vi "Retrieve CD dependencies from properties.vi"(11 "main page properties in":T5) -> (2 "custom device dependencies":T1[](array[typedef]), 3 "main page properties out":T5)   [LabVIEW 2019, in "HLA Custom Device System Explorer.lvlib"]
uses:
  HLA Custom Device System Explorer.lvlib
  Shared/main_page_config.ctl
  <vilib>/NI VeriStand/Custom Device API/Custom Device File Dependency.ctl
  <vilib>/NI VeriStand/Custom Device API/Path Specification.ctl
  <vilib>/NI VeriStand/Custom Device API/Path Type.ctl
  <vilib>/NI VeriStand/Custom Device API/Custom Device Supported Target.ctl
  Shared/HLA Custom Device Shared.lvlib
  <vilib>/NI VeriStand/Custom Device API/Custom Device API.lvlib
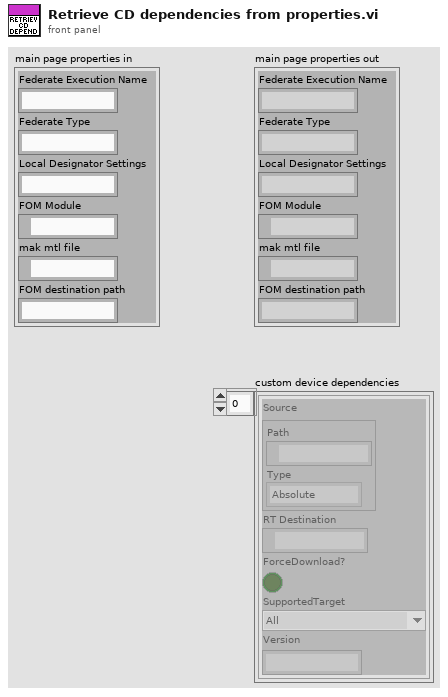
[diagram p1: front panel]
types:
  T1 = typedef "Custom Device API.lvlib/Custom Device File Dependency.ctl" = cluster{"Source":T2, "RT Destination":path, "ForceDownload?":bool, "SupportedTarget":T4, "Version":string}
  T2 = typedef "Custom Device API.lvlib/Path Specification.ctl" = cluster{"Path":path, "Type":T3}
  T3 = typedef "Custom Device API.lvlib/Path Type.ctl" = enum16{"Absolute", "To Base", "To Common Data Dir", "To Application Data Dir"}
  T4 = typedef "Custom Device API.lvlib/Custom Device Supported Target.ctl" = enum16{"All", "PharLap", "VxWorks", "Windows", "Linux_32_ARM", "Linux_x64", "PharLap & Windows", "PharLap & VxWorks", "VxWorks & Windows"}
  T5 = typedef "HLA Custom Device Shared.lvlib/main_page_config.ctl" = cluster{"Federate Execution Name":string, "Federate Type":string, "Local Designator Settings":string, "FOM Module":path, "mak mtl file":path, "FOM destination path":string}
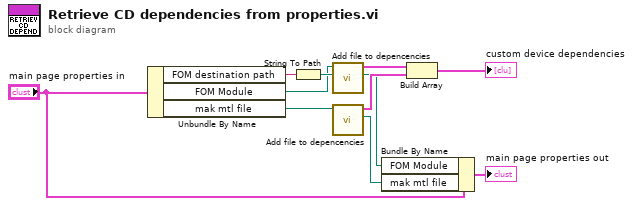
[diagram p0: block diagram]
diagram:
  n1 = Unbundle By Name("main page properties in") -> ("FOM destination path"=w11:string, "FOM Module"=w1:path, "mak mtl file"=w9:path)
  n2 = String To Path(string=w11) -> (path=w10:path)
  n3 = call "Add file to depencencies.vi"("RT Destination folder (c:\\ni-rt\\NIVeriStand)"=w10, "item path"=w1) -> ("destination path"=w6:path, "dependency out"=w2:T1)  [unwired: 8 in]
  n4 = call "Add file to depencencies.vi"("item path"=w9) -> ("destination path"=w7:path, "dependency out"=w8:T1)  [unwired: 9 in]
  n5 = Bundle By Name(cluster="main page properties in", "FOM Module"=w6, "mak mtl file"=w7) -> (→"main page properties out":T5)
  n6 = Build Array(w2, w8) -> (→"custom device dependencies":T1[])
